vi "Configure CAN.vi"(8 "error in":errorcluster, 11 "HSU MCU V2 Monitor CFG in":refnum<class "HSU MCU V2 CFG.lvclass">) -> (0 "error out":errorcluster, 3 "HSU MCU V2 Monitor CFG out":refnum<class "HSU MCU V2 CFG.lvclass">)   [LabVIEW 2023, in "HSU MCU V2 CFG.lvclass"]
uses:
  HSU MCU V2 CFG.lvclass
  HSU MCU V2 CFG.lvclass/HSU MCU V2 CFG.ctl
  Protocols/ICAN/ICAN.lvclass
  <vilib>/JDP Science/JSONtext/JSONtext.lvlib
  Configurations/CFG JSON/CFG JSON.lvclass
  60c77de9-abfb-4302-865d-68a0323ddca5.vi
  D:/git/HAL/HAL/Configurations/CFG JSON/CFG JSON.lvclass
  D:/git/HAL/HAL/Configurations/CFG Base/CFG Base.lvclass
  D:/git/HAL/HAL/Devices/HSU MCU V2 CFG/HSU MCU V2 CFG.lvclass
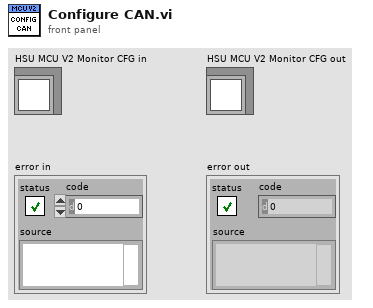
[diagram p1: front panel]
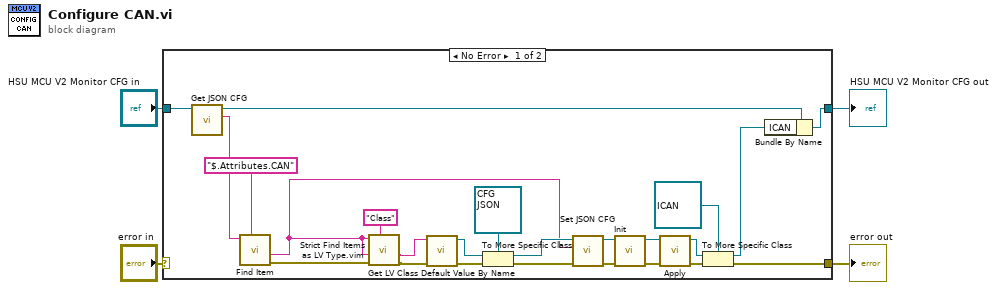
[diagram p0: block diagram]
diagram:
  n1 = case shown="No Error" "error in" {
    selector: "error in" -> [_ w29]
    tunnel: [w18 w29] -> w3
    tunnel: [w25 w28] -> w1
    tunnel: "HSU MCU V2 Monitor CFG in" -> [w27 w28]
    frame No Error {
      n2 = call "Get JSON CFG.vi"("CFG JSON in"=w27) -> ("<JSON> CFG"=w11:string, "CFG JSON out"=w26:refnum<class "HSU MCU V2 CFG.lvclass">)  [unwired: 9 in]
      n3 = call <vilib>:"Find Item.vi"("$Path or Item Name"="$.Attributes.CAN", "JSON"=w11) -> ("error out"=w10:errorcluster, "<JSON>"=w9:string)  [unwired: 6 in, 2 out]
      n4 = call "Strict Find Items as LV Type.vim"("$Path or Item Name"="Class", "error in"=w10, "Data Type and Default Value"=w9, "<JSON>"=w9) -> ("error out"=w6:errorcluster, "Data out"=w7:string)  [unwired: 5 in, 1 out]
      n5 = call <vilib>:"Get LV Class Default Value By Name.vi"("error in (no error)"=w6, "class name"=w7) -> ("error out"=w24:errorcluster, "object"=w22:refnum<class>)  [unwired: 8 in]
      n6 = To More Specific Class(target class=refnum<class "CFG JSON.lvclass"> refnum ("ICommunicate.lvclass"), reference=w22, error in=w24) -> (specific class reference=w13:refnum<class "CFG JSON.lvclass">, error out=w5:errorcluster)
      n7 = call "Set JSON CFG.vi"("<JSON> CFG"=w9, "CFG JSON in"=w13) -> ("CFG JSON out"=w14:refnum<class "CFG JSON.lvclass">)  [unwired: 9 in]
      n8 = call-dynamic "Init.vi"("error in"=w5, "CFG Base in"=w14) -> ("error out"=w21:errorcluster, "CFG Base out"=w19:refnum<class "CFG JSON.lvclass">)  [unwired: 8 in]
      n9 = call-dynamic "Apply.vi"("error in"=w21, "CFG Base in"=w19) -> ("error out"=w20:errorcluster, "CFG Base out"=w17:refnum<class "CFG JSON.lvclass">)  [unwired: 8 in]
      n10 = To More Specific Class(target class=refnum<class "ICAN.lvclass"> refnum ("ICAN.lvclass"), reference=w17, error in=w20) -> (specific class reference=w15:refnum<class "ICAN.lvclass">, error out=w18:errorcluster)
      n11 = Bundle By Name(cluster=w26, "ICAN"=w15) -> (w25:refnum<class "HSU MCU V2 CFG.lvclass">)
    }
    frame Error {
    }
  }
  "error out" <- w3
  "HSU MCU V2 Monitor CFG out" <- w1
